vi "FreshScroll.vi"(8 "error in (no error)":errorcluster, 11 "AdvanceTable in":refnum<class "AdvanceTable.lvclass">) -> (0 "error out":errorcluster, 3 "AdvanceTable out":refnum<class "AdvanceTable.lvclass">)   [LabVIEW 2015, in "ActorManagement.lvlib" / "AdvanceTable.lvclass"]
uses:
  AdvanceTable.lvclass
  AdvanceTable.lvclass/AdvanceTable.ctl
  Scroll/Scroller.lvclass
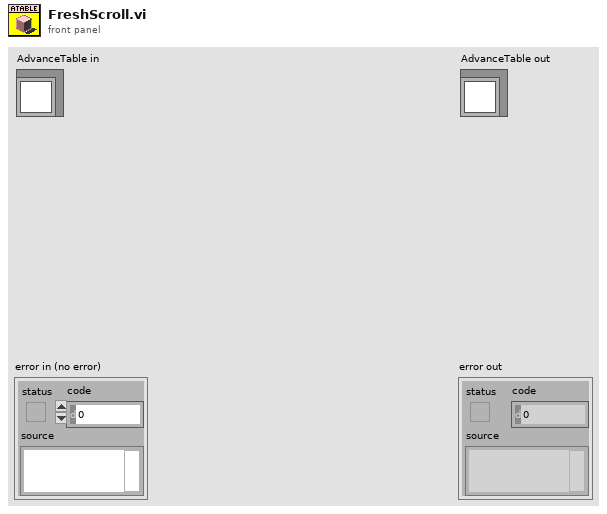
[diagram p1: front panel]
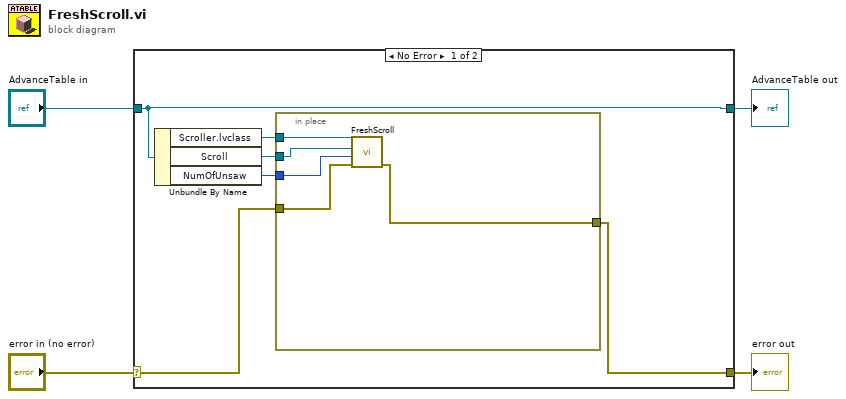
[diagram p0: block diagram]
diagram:
  n1 = case shown="No Error" "error in (no error)" {
    selector: "error in (no error)" -> [w6 w17]
    tunnel: [w5 w17] -> w3
    tunnel: [w10 w16] -> w1
    tunnel: "AdvanceTable in" -> [w10 w16]
    frame No Error {
      n2 = Unbundle By Name(w10) -> ("Scroller.lvclass"=w7:refnum<class "Scroller.lvclass">, "Scroll"=w8:refnum<vi>, "NumOfUnsaw"=w9:u32)
      n3 = in-place {
        in-place-border: w9 -> [w11]
        in-place-border: w8 -> [w14]
        in-place-border: w7 -> [w15]
        in-place-border: w6 -> [w13]
        in-place-border: [w12] -> w5
        n4 = call "FreshScroll.vi"("error in (no error)"=w13, "Index"=w11, "Scroll"=w14, "Scroller.lvclass"=w15) -> ("error out"=w12:errorcluster)  [unwired: 6 in, 1 out]
      }
    }
    frame Error {
    }
  }
  "error out" <- w3
  "AdvanceTable out" <- w1
